vi "Test.vi"() -> ()   [LabVIEW 2017]
uses:
  Crabtree LAB Panel/Lab Panel V2/program files/Global 1.vi
panel:
  out "Zero Counters":u64[](array[numeric])
  in  "stop":bool
  out "LA05 TEMP":T1
  out "LA04 TEMP":T1
  out "LA03 TEMP":T1
  out "LA02 TEMP":T1
  out "LA01 TEMP":T1
  out "Com Port Status":bool
  out "Com setup loops":i32
  out "VISA Com out":refnum<visa-resource-name>
  in  "Select COM port":refnum<visa-resource-name>="COM6"
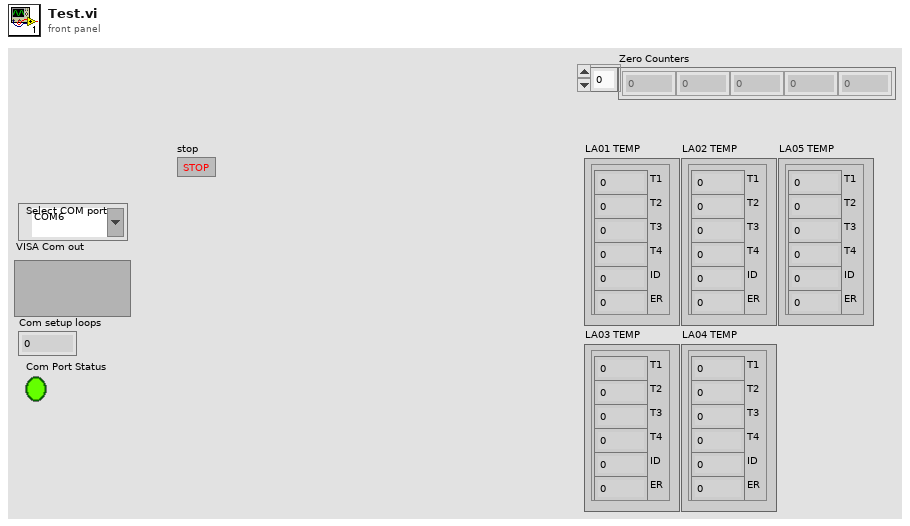
[diagram p1: front panel]
types:
  T1 = cluster{"T1":dbl, "T2":dbl, "T3":dbl, "T4":dbl, "ID":dbl, "ER":dbl}
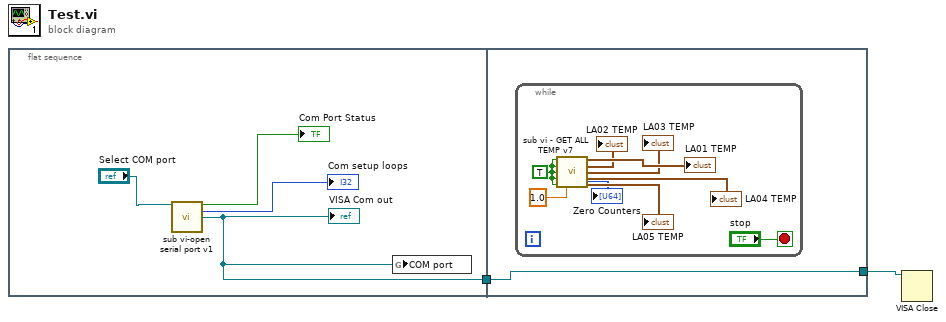
[diagram p0: block diagram]
diagram:
  n1 = flat-sequence {
    tunnel: [w3] -> w2
    tunnel: [w7] -> _
    tunnel: w2 -> [w7]
    tunnel: [w7] -> w1
    frame #0 {
      n2 = call "sub vi-open serial port v1.vi"("Select COM port"="Select COM port") -> ("Error"=→"Com Port Status":bool, "LOOPS"=→"Com setup loops":i32, "VISA Com out"=w3:refnum<visa-resource-name>)  [unwired: 12 in]
      "VISA Com out" <- w3
      n3 = global write "Global 1.vi" "COM port"(w3) -> ()
    }
    frame #1 {
      n4 = while {
        stop <- "stop" stop-if-true
        w16 = TRUE ("LA03-EN")
        n5 = call "sub vi - GET ALL TEMP v7.vi"("LA01-EN"=w16, "LA02-EN"=w16, "LA03-EN"=w16, "LA04-EN"=w16, "LA05-EN"=w16, "Gen Cal Value"=1.0) -> ("LA01 TEMP"=→"LA01 TEMP":T1, "LA02 TEMP"=→"LA02 TEMP":T1, "LA03 TEMP"=→"LA03 TEMP":T1, "LA04 TEMP"=→"LA04 TEMP":T1, "Zero Counters"=→"Zero Counters":u64[], "LA05 TEMP"=→"LA05 TEMP":T1)  [unwired: 1 in, 3 out]
      }
    }
  }
  n6 = VISA Close(VISA resource name=w1) -> ()  [unwired: 1 in, 1 out]
